vi "battery.vi"(7 "LabVIEW Web Service Request":refnum<class "Web Request.lvclass">) -> (2 "state":string, 3 "voltage":string)   [LabVIEW 2014]
uses:
  <vilib>/wsapi/Web Request.lvclass
  DronePi Global Variables.vi
panel:
  # "Use the Web Service Request input terminal to call the VIs on the Web Services palette. Do not remove it from the connector pane unless you don't need access to the palette."
  # "Each additional control wired to the connector pane will be available as an input in the URL. To include an indicator in terminal-mode output (the default setting), it must also be wired to the connector pane."
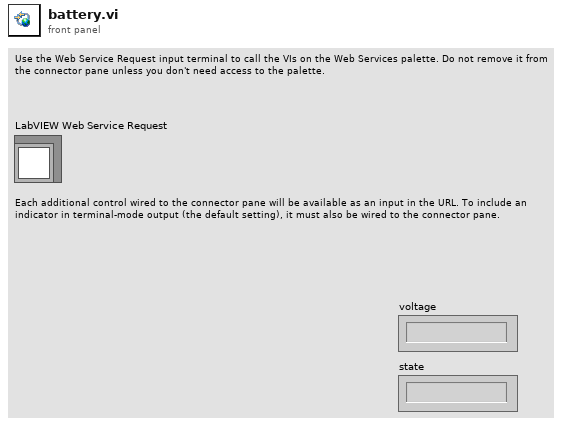
[diagram p1: front panel]
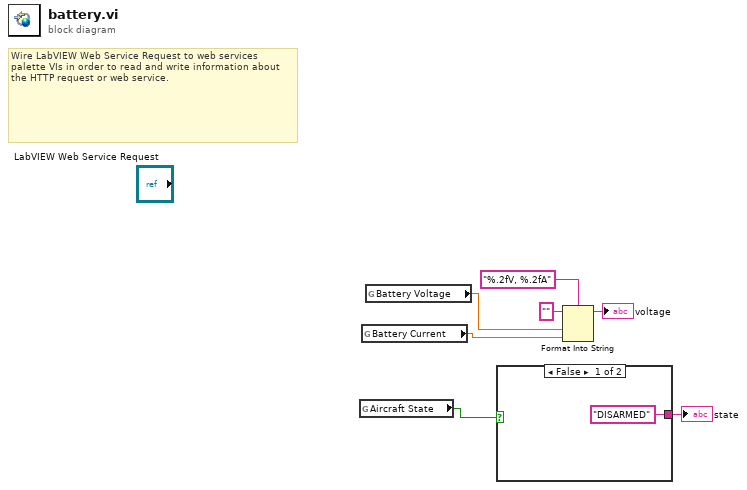
[diagram p0: block diagram]
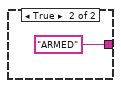
[diagram p2: hidden frame]
diagram:
  # "Wire LabVIEW Web Service Request to web services palette VIs in order to read and write information about the HTTP request or web service."
  n1 = global read "DronePi Global Variables.vi" "Aircraft State"() -> (w2:bool)
  n2 = global read "DronePi Global Variables.vi" "Battery Current"() -> (w6:dbl)
  n3 = global read "DronePi Global Variables.vi" "Battery Voltage"() -> (w7:dbl)
  n4 = case shown="False" w2 {
    tunnel: ["DISARMED" "ARMED"] -> w1
    frame False {
    }
    frame True {
    }
  }
  "state" <- w1
  n5 = Format Into String(format string="%.2fV, %.2fA", initial string="", w7, w6) -> (resulting string=→"voltage":string)  [unwired: 1 in, 1 out]
